vi "ConvertWaveformsToAmplitudeSpectra.vi"(5 "Averaging Mode":T3(ring), 6 "Number of Averages":dbl, 7 "Weighting Mode":enum16{"Linear", "Exponential"}(ring), 8 "Export Mode":T1 items=["Power Spectrum", "Power Spectral Density"], 9 "Waveforms":waveform(dbl)[](array[waveform]), 10 "Window":T2=1 items=["Rectangle"=0, "Hanning"=1, "Hamming"=2, "Blackman-Harris"=3, "Exact Blackman"=4, "Blackman"=5, "Flat Top"=6, "4 Term B-Harris "=7, "7 Term B-Harris"=8, "Low Sidelobe"=9, "Blackman Nuttall"=11, "Triangle"=30, "Bartlett-Hanning"=31, "Bohman"=32, "Parzen"=33, "Welch"=34, "Kaiser"=60, "Dolph-Chebyshev"=61, "Gaussian"=62], 11 "Restart Averaging":bool) -> (0 "Frequency Resolution [Hz]":dbl, 1 "Amplitude Spectral Density":cluster{"f0":dbl, "df":dbl, "magnitude":dbl[]}[](array[cluster]), 2 "Averages Completed":dbl, 3 "Averaging Done":bool, 4 "ENBW [Hz]":dbl)   [LabVIEW 2020]
uses:
  <vilib>/Analysis/4window.llb/windowTd.ctl
  <vilib>/measure/maspectr.llb/Power Spectrum and PSD Export Mode.ctl
  <vilib>/Analysis/0measdsp.llb/Scaled Time Domain Window (DBL).vi
  <vilib>/measure/maspectr.llb/FFT Power Spectrum and PSD for N Chan.vi
  <vilib>/measure/NI_MAPro.lvlib
  <vilib>/Analysis/NI_AALPro.lvlib
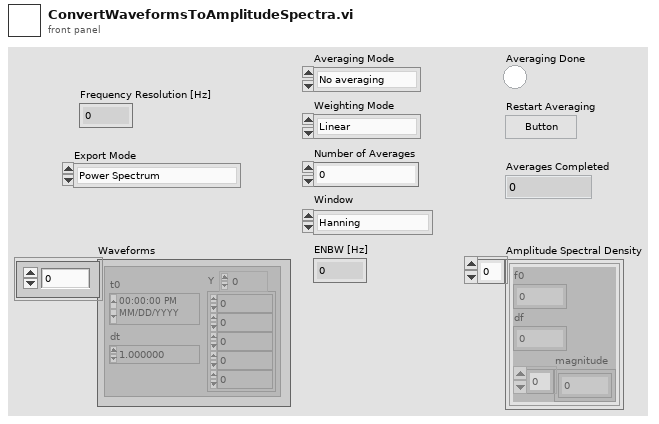
[diagram p1: front panel]
types:
  T1 = typedef "NI_MAPro.lvlib/Power Spectrum and PSD Export Mode.ctl" = u16
  T2 = typedef "NI_AALPro.lvlib/windowTd.ctl" = u32
  T3 = enum16{"No averaging", "Vector averaging", "RMS averaging", "Peak hold"}
  T4 = cluster{"averaging mode":enum16{"No averaging", "Vector averaging", "RMS averaging", "Peak hold"}, "weighting mode":enum16{"Linear", "Exponential"}, "number of averages":u32}
  T5 = cluster{"Power Spectrum / PSD[0]":cluster{"f0":dbl, "df":dbl, "magnitude":dbl[]}, "Power Spectrum / PSD[1]":cluster{"f0":dbl, "df":dbl, "magnitude":dbl[]}, "Power Spectrum / PSD[2]":cluster{"f0":dbl, "df":dbl, "magnitude":dbl[]}, "Power Spectrum / PSD[3]":cluster{"f0":dbl, "df":dbl, "magnitude":dbl[]}, "Power Spectrum / PSD[4]":cluster{"f0":dbl, "df":dbl, "magnitude":dbl[]}, "Power Spectrum / PSD[5]":cluster{"f0":dbl, "df":dbl, "magnitude":dbl[]}, "Power Spectrum / PSD[6]":cluster{"f0":dbl, "df":dbl, "magnitude":dbl[]}, "Power Spectrum / PSD[7]":cluster{"f0":dbl, "df":dbl, "magnitude":dbl[]}, "Power Spectrum / PSD[8]":cluster{"f0":dbl, "df":dbl, "magnitude":dbl[]}}
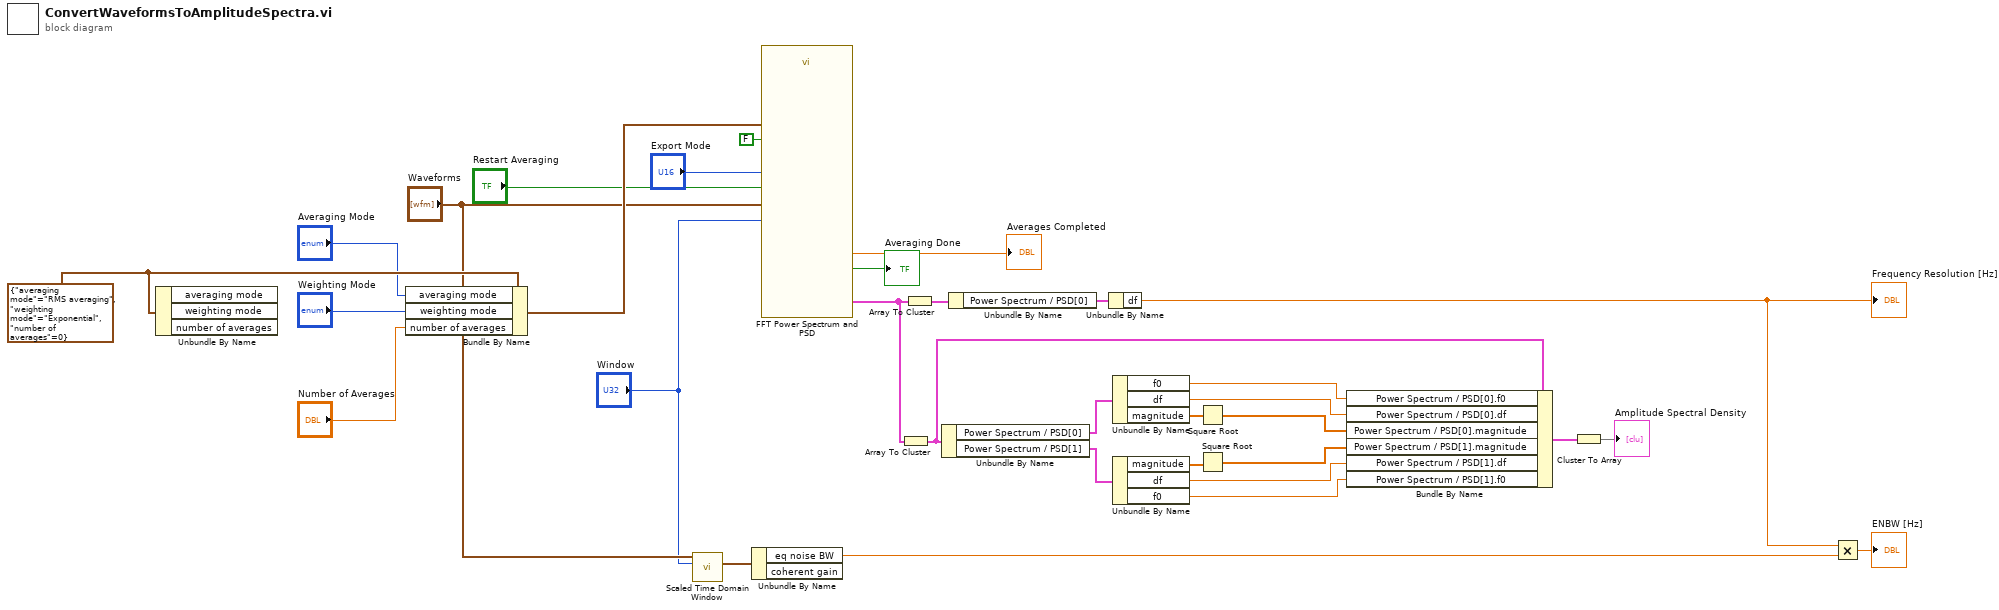
[diagram p0: block diagram]
diagram:
  w32 = T4 {"averaging mode"=enum."RMS averaging", "weighting mode"=enum."Exponential", "number of averages"=0} ("averaging parameters")
  n1 = Unbundle By Name(w32) -> ()  [unwired: 3 out]
  n2 = Bundle By Name(cluster=w32, "averaging mode"="Averaging Mode", "weighting mode"="Weighting Mode", "number of averages"="Number of Averages") -> (w30:T4)
  n3 = call-poly <vilib>:"Scaled Time Domain Window.vi"("window"="Window", "X"="Waveforms") -> ("window properties"=w6:cluster{"eq noise BW":dbl, "coherent gain":dbl})  [unwired: 7 in, 2 out]
  n4 = Unbundle By Name(w6) -> ("eq noise BW"=w1:dbl)  [unwired: 1 out]
  n5 = call-poly <vilib>:"FFT Power Spectrum and PSD.vi"("export mode"="Export Mode", "averaging parameters"=w30, "restart averaging (F)"="Restart Averaging", "dB On (F)"=FALSE, "window"="Window", "time signals"="Waveforms") -> ("averages completed"=→"Averages Completed":dbl, "averaging done"=→"Averaging Done":bool, "Power Spectrum / PSD"=w23:cluster{"f0":dbl, "df":dbl, "magnitude":dbl[]}[])  [unwired: 2 in, 1 out]
  n6 = Array To Cluster(array=w23) -> (cluster=w19:T5)
  n7 = Array To Cluster(array=w23) -> (cluster=w25:T5)
  n8 = Unbundle By Name(w19) -> ("Power Spectrum / PSD[0]"=w20:cluster{"f0":dbl, "df":dbl, "magnitude":dbl[]}, "Power Spectrum / PSD[1]"=w22:cluster{"f0":dbl, "df":dbl, "magnitude":dbl[]})
  n9 = Unbundle By Name(w25) -> ("Power Spectrum / PSD[0]"=w24:cluster{"f0":dbl, "df":dbl, "magnitude":dbl[]})
  n10 = Unbundle By Name(w24) -> ("df"=w2:dbl)
  "Frequency Resolution [Hz]" <- w2
  n11 = Unbundle By Name(w20) -> ("f0"=w10:dbl, "df"=w13:dbl, "magnitude"=w17:dbl[])
  n12 = Unbundle By Name(w22) -> ("magnitude"=w16:dbl[], "df"=w12:dbl, "f0"=w11:dbl)
  n13 = Square Root(x=w17) -> (sqrt(x)=w15:dbl[])
  n14 = Square Root(x=w16) -> (sqrt(x)=w14:dbl[])
  n15 = Bundle By Name(cluster=w19, "Power Spectrum / PSD[0].f0"=w10, "Power Spectrum / PSD[0].df"=w13, "Power Spectrum / PSD[0].magnitude"=w15, "Power Spectrum / PSD[1].magnitude"=w14, "Power Spectrum / PSD[1].df"=w12, "Power Spectrum / PSD[1].f0"=w11) -> (w18:T5)
  n16 = Cluster To Array(cluster=w18) -> (array=→"Amplitude Spectral Density":cluster{"f0":dbl, "df":dbl, "magnitude":dbl[]}[])
  n17 = Multiply(x=w2, y=w1) -> (x*y=→"ENBW [Hz]":dbl)
